vi "WSVCAP SHL Host LL I2C Build and Parse Read Message.vi"(0 "C1 Read Data In":u8[][](array[numeric]) format="%.0x", 1 "Message In":string, 11 "error in":errorcluster, 12 "Status In":u8[](array[numeric])) -> (3 "Message Out":string, 4 "C1 Read Data Out":u8[][](array[numeric]) format="%.0x", 14 "Status":u8[](array[numeric]), 15 "error out":errorcluster)   [LabVIEW 2017]
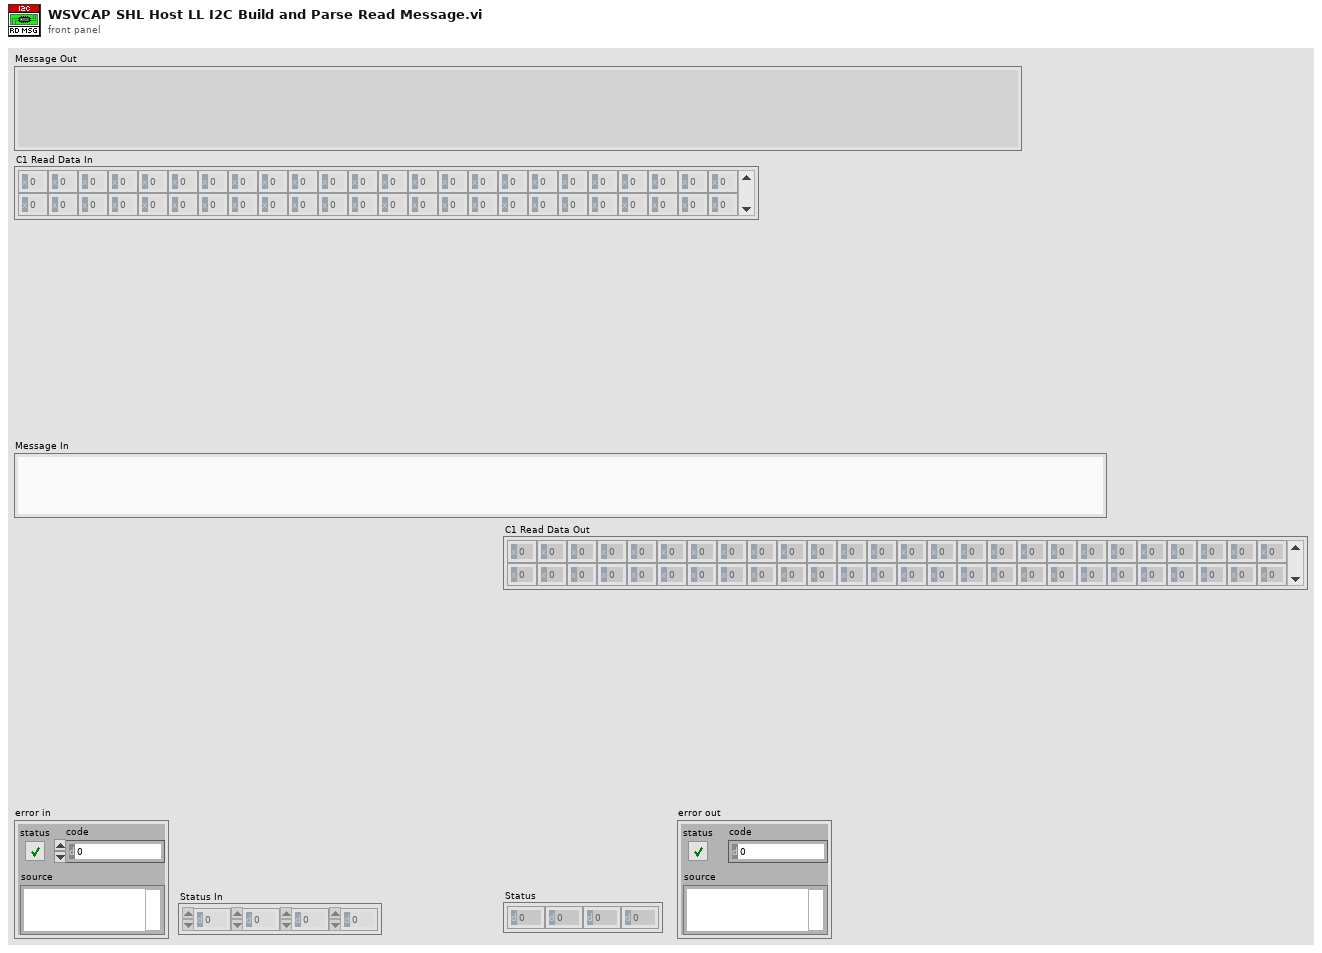
[diagram p1: front panel]
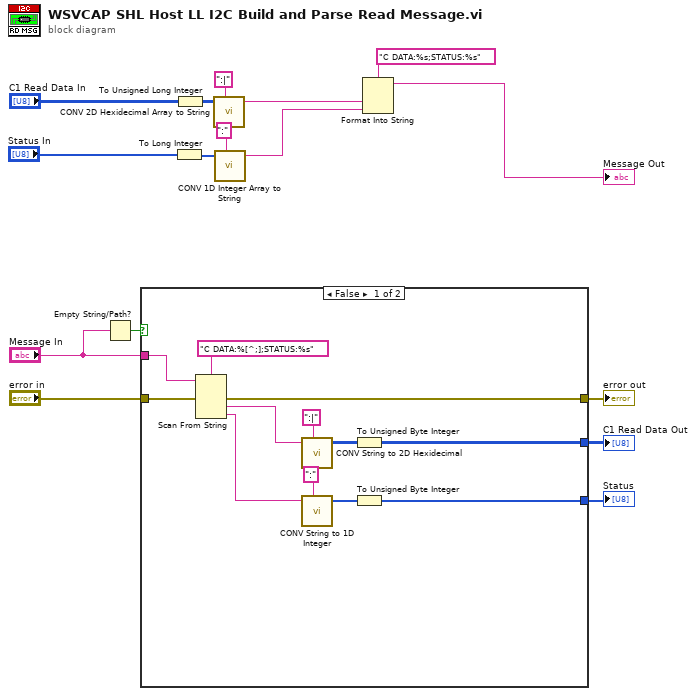
[diagram p0: block diagram]
diagram:
  n1 = Empty String/Path?(string/path="Message In") -> (empty?=w5:bool)
  n2 = case shown="False" w5 {
    tunnel: [w27 _] -> w13
    tunnel: "error in" -> [w24 w29]
    tunnel: [w20 _] -> w8
    tunnel: "Message In" -> [w18 _]
    tunnel: [w19 w29] -> w4
    frame False {
      n3 = Scan From String(format string="C DATA:%[^;];STATUS:%s", input string=w18, error in=w24) -> (error out=w19:errorcluster, output 1=w25:string, output 2=w23:string)  [unwired: 3 in, 2 out]
      n4 = call "CONV String to 2D Hexidecimal.vi"("String"=w25, "Delimiters (,;)"=":|") -> ("2-D Hexidecimal"=w28:u32[][])  [unwired: 7 in]
      n5 = call "CONV String to 1D Integer.vi"("String"=w23, "Delimiter (,)"=":" ("Delimiters (,;)")) -> ("1-D Integer"=w21:i32[])  [unwired: 7 in]
      n6 = To Unsigned Byte Integer(number=w28) -> (unsigned 8bit integer=w27:u8[][])
      n7 = To Unsigned Byte Integer(number=w21) -> (unsigned 8bit integer=w20:u8[])
    }
    frame True {
    }
  }
  "C1 Read Data Out" <- w13
  "error out" <- w4
  "Status" <- w8
  n8 = To Long Integer(number="Status In") -> (32bit integer=w10:i32[])
  n9 = To Unsigned Long Integer(number="C1 Read Data In") -> (unsigned 32bit integer=w16:u32[][])
  n10 = call "CONV 2D Hexidecimal Array to String.vi"("2-D Hexidecimal"=w16, "Delimiters (,;)"=":|") -> ("String"=w15:string)  [unwired: 7 in]
  n11 = call "CONV 1D Integer Array to String.vi"("1-D Integer"=w10, "Delimiter (,)"=":" ("Delimiters (,;)")) -> ("String"=w9:string)  [unwired: 7 in]
  n12 = Format Into String(format string="C DATA:%s;STATUS:%s", w15, w9) -> (resulting string=→"Message Out":string)  [unwired: 2 in, 1 out]
